vi "Initialize.vi"(8 "error in (no error)":errorcluster caption="错误输入（无错误）", 11 "Channel输入":refnum<class "Channel.lvclass">) -> (0 "error out":errorcluster caption="错误输出", 3 "Channel输出":refnum<class "Channel.lvclass">)   [LabVIEW 2013, in "Hierarchy Framework.lvlib" / "Channel.lvclass"]
uses:
  Channel.lvclass
  Item/Item.lvclass
  Channel.lvclass/Channel.ctl
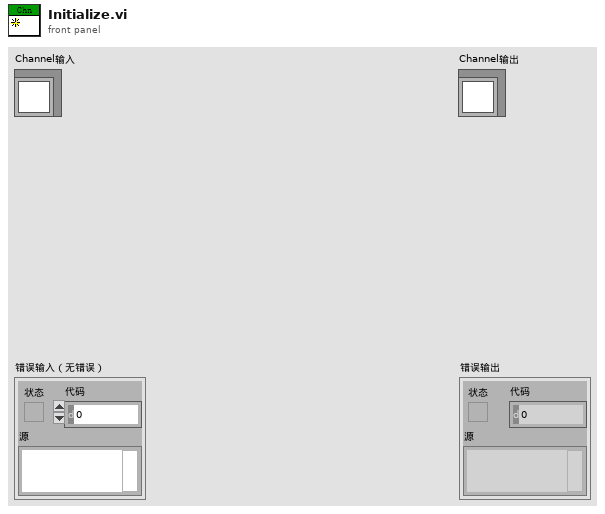
[diagram p1: front panel]
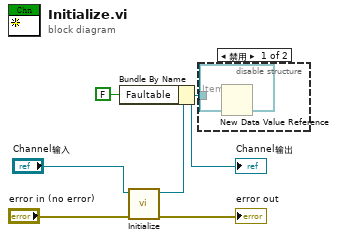
[diagram p0: block diagram]
diagram:
  n1 = call-parent "Initialize.vi"("error in (no error)"="error in (no error)", "Item输入"="Channel输入") -> ("error out"=→"error out":errorcluster, "Item输出"=w2:refnum<class "Channel.lvclass">)  [unwired: 8 in]
  n2 = Bundle By Name(cluster=w2, "Faultable"=FALSE) -> (w1:refnum<class "Channel.lvclass">)
  "Channel输出" <- w1
  n3 = disable-structure shown="禁用" {
    disable-tunnel: w1 -> [w7 _]
    frame Disabled {
      (unwired) refnum<data-value> refnum ("数据值引用")
      n4 = New Data Value Reference(data value=w7) -> ()  [unwired: 1 in, 2 out]
    }
    frame Enabled {
    }
  }
